vi "_Open VI FP.vi"() -> ()   [LabVIEW 2014]
panel:
  in  "vi path":path
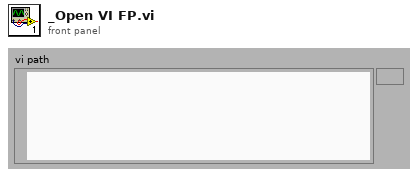
[diagram p1: front panel]
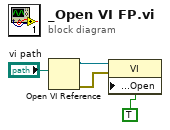
[diagram p0: block diagram]
diagram:
  n1 = Open VI Reference(vi path="vi path") -> (vi reference=w3:refnum<vi>, error out=w2:errorcluster)  [unwired: 5 in]
  n2 = property class="VI"(reference=w3, error in=w2, "Front Panel.Open"=TRUE) -> ()  [unwired: 2 out]
